vi "Compiled Settings Name.vi"(11 "CD Template in":refnum<class "NIVS_PPL_Inline HW Interface (Inline-Async).lvclass">) -> (2 "Compiled Settings Name":string)   [LabVIEW 2019, in "NIVS_PPL_Inline HW Interface (Inline-Async).lvclass"]
uses:
  NIVS_PPL_Inline HW Interface (Inline-Async).lvclass
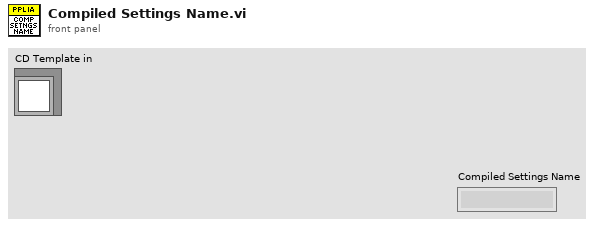
[diagram p1: front panel]
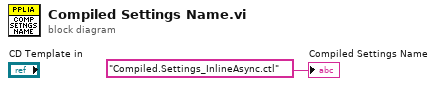
[diagram p0: block diagram]
diagram:
  "Compiled Settings Name" <- "Compiled.Settings_InlineAsync.ctl" ("Compiled Settings Name")
